vi "Main menu_4.vi"() -> ()   [LabVIEW 2021]
uses:
  <vilib>/event_ctls.llb/lveventtype.ctl
  <vilib>/Utility/file.llb/Write Delimited Spreadsheet (DBL).vi
panel:
  in  "Clear error":bool
  out "Error":bool
  out "Close":bool
  in  "?":T1(tab)
  in  "New_plot_window":bool
  in  "List of active windows":i32(listbox)
  in  "Close All plots":bool
  out "Trace_total samples":i32
  in  "CSV":bool
  in  "Start record":bool
  in  "Refresh \ntime (ms)":i32
  in  "Global Mode":enum32{"Item 0", "Item 1"}(radio)
  in  "Samples X Signal":u32
  in  "Trace names":string(combo)
  out "Signals":i32
  in  "CTRL enable":bool
  in  "Save CTRL parameters":bool
  out "Total\ncontrols":i32
  in  "# Control":string(combo)
  in  "CS enable":bool
  out "Current CS status":i32
  in  "CS_IF_Params":T2 {"CS_Duty" min=0 max=1}
  out "Connected":bool
  out "Saved":bool
  in  "Save conf":bool
  in  "Port":i32
  in  "hostname":string
  in  "timeout ms":i32
  in  "Send message":bool
  in  "Process":i32
  in  "msj":string
  out "error out":errorcluster
  # "ctrl_if:0\nctrl: 2\nset parm: 2"
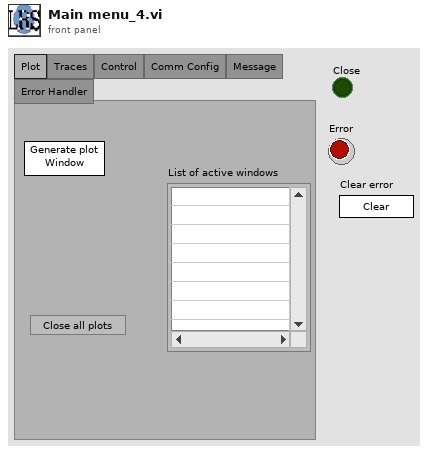
[diagram p1: front panel]
types:
  T1 = enum32{"Plot", "Traces", "Control", "Comm Config", "Message", "Error Handler"}
  T2 = cluster{"SET_PARAMETERS":i32, "CTLR":i32, "CS_Duty":sgl, "CTRL_IF_SET":i32}
  T3 = cluster{"Port":i32, "hostname":string, "status":bool, "timeout ms":i32, "TRACES_NAMES":string[], "Refresh time ms":i32, "Mode":enum32{"Item 0", "Item 1"}, "Start":bool, "DATA":sgl[][], "SIGNALS_NAMES":string[], "NB_SIGNALS":i32, "NB_TRACES":i32, "ID_TRACE":i32, "Mark":bool, "Counter":i32, "CTRLs_NAMES":string[], "NB_Ctrls":i32, "CS enable?":bool, "CS ID":i32}
  T4 = enum8{"Enabled", "Disabled", "Disabled and Grayed Out"}
  T5 = typedef "lveventtype.ctl" = enum32{"Null", "Timeout", "Annotation Menu Selection", "Annotation Menu Selection?", "App Instance Close", "App Instance Close?", "Autoscale Range Change", "Bookmark Info Change", "Cell Edit", "Cell Edit?", "Cursor Grab", "Cursor Grab?", "Cursor Menu Selection", "Cursor Menu Selection?", "Cursor Move", "Cursor Release", "Data Change", "Direction Change", "Display State Change", "Drag Ended", "Drag Enter", "Drag Leave", "Drag Over", "Drag Source Update", "Drag Starting", "Drag Starting?", "Drop", "Exec State Change", "Key Down", "Key Down?", "Key Repeat", "Key Repeat?", "Key Up", "Listbox Double Click", "Menu Activation?", "Menu Selection (App)", "Menu Selection? (App)", "Menu Selection (User)", "Mouse Down", "Mouse Down?", "Mouse Enter", "Mouse Leave", "Mouse Move", "Mouse Up", "Mouse Wheel", "NI Security User Change (App)", "Pane Size", "Panel Close", "Panel Close?", "Panel Resize", "Plot Attribute Change", "Scale Range Change", "Shortcut Menu Activation?", "Shortcut Menu Selection (App)", "Shortcut Menu Selection? (App)", "Shortcut Menu Selection (User)", "Tree Double Click", "Tree Drag", "Tree Drag?", "Tree Drop", "Tree Drop?", "Tree Item Close", "Tree Item Close?", "Tree Item Open", "Tree Item Open?", "User Event", "Value Change"}
  T6 = enum16{"open", "replace", "create", "open or create", "replace or create", "replace or create with confirmation"}
  T7 = enum32{"Invalid", "Standard", "Closed", "Hidden", "Minimized", "Maximized"}
  T8 = enum32{"invalid app kind", "Development System", "Run Time System", "Student Edition", "Embedded LabVIEW", "Evaluation", "Custom"}
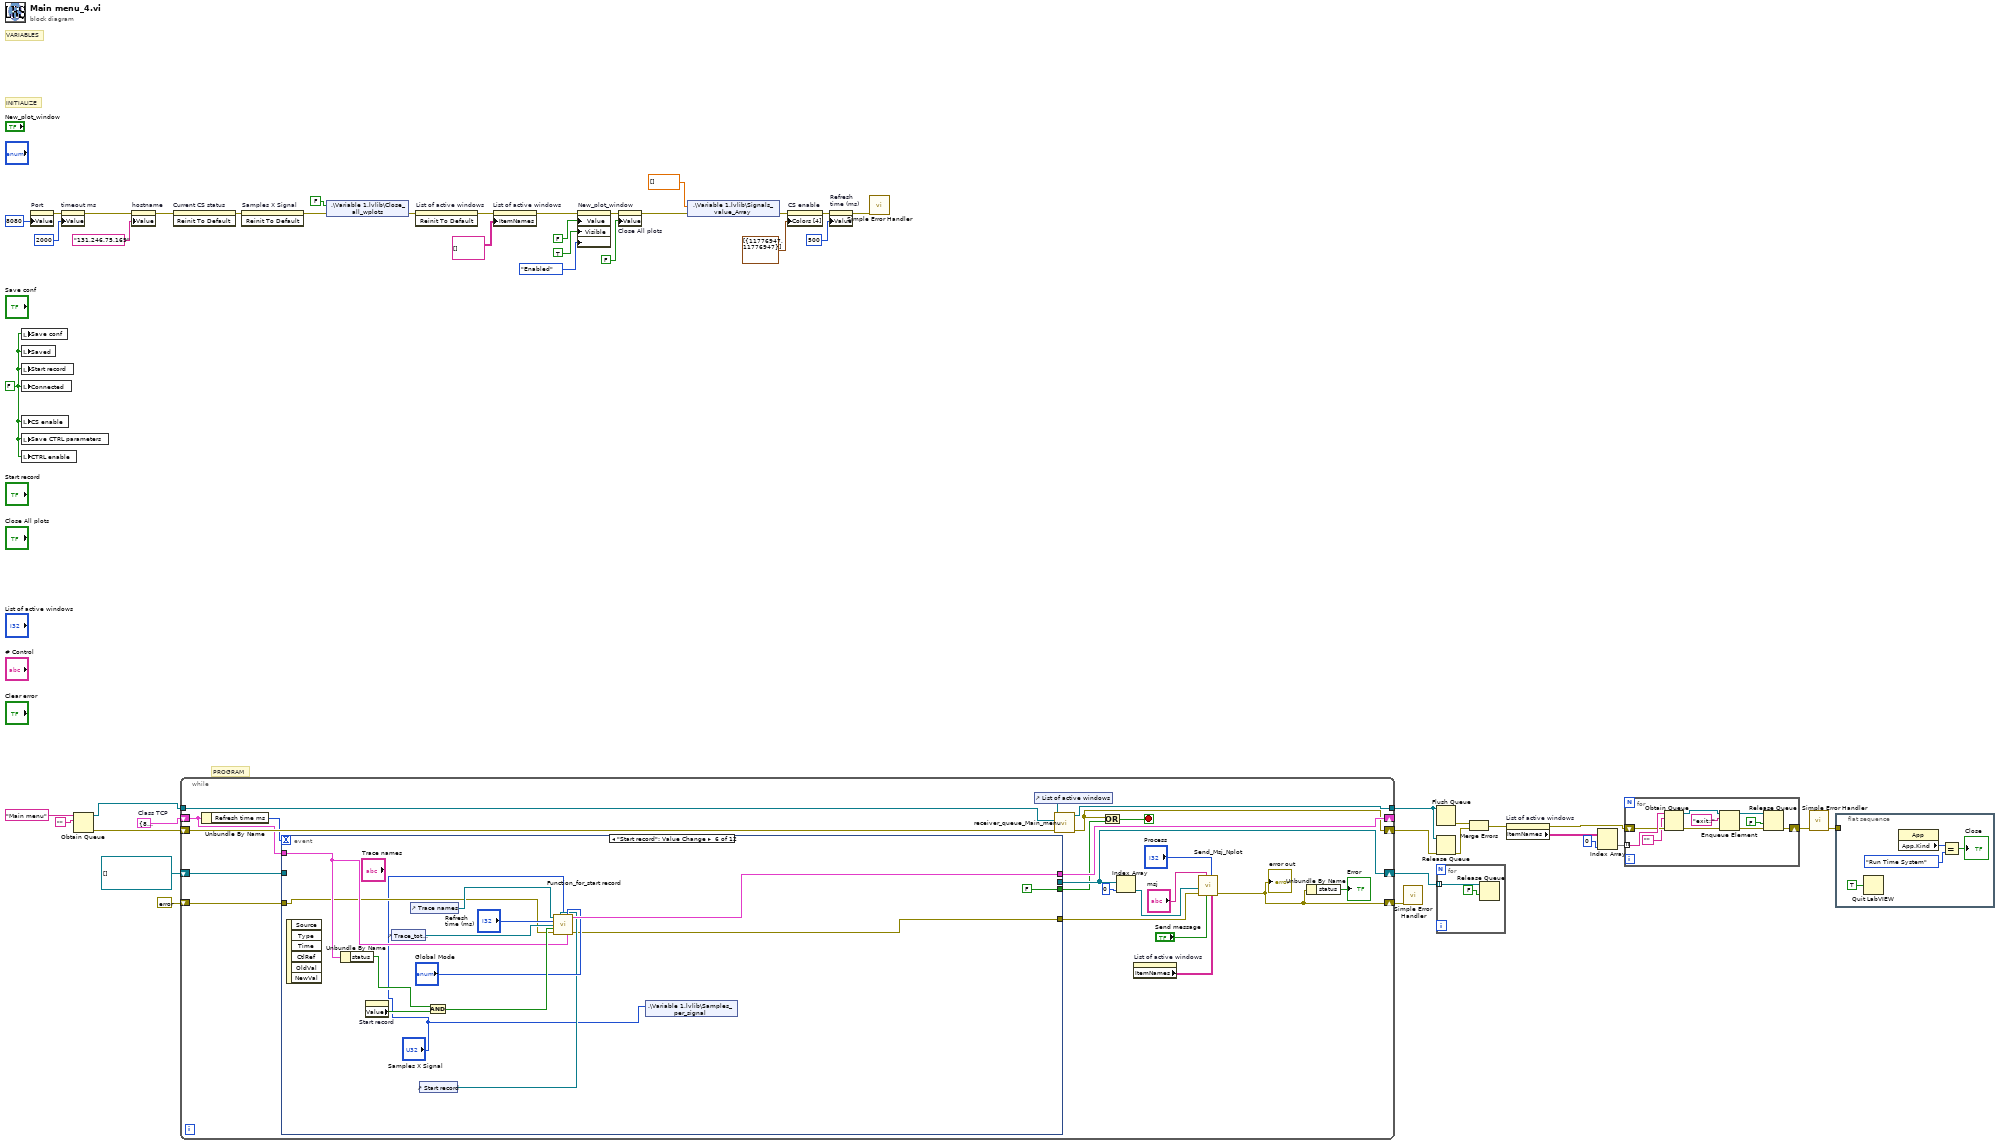
[diagram p0: block diagram]
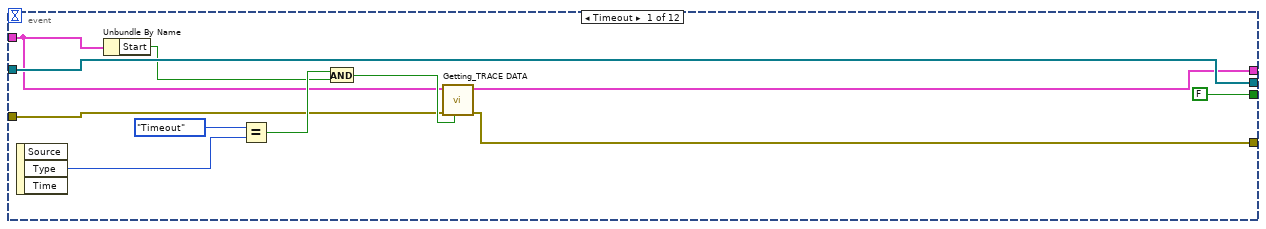
[diagram p2: hidden frame]
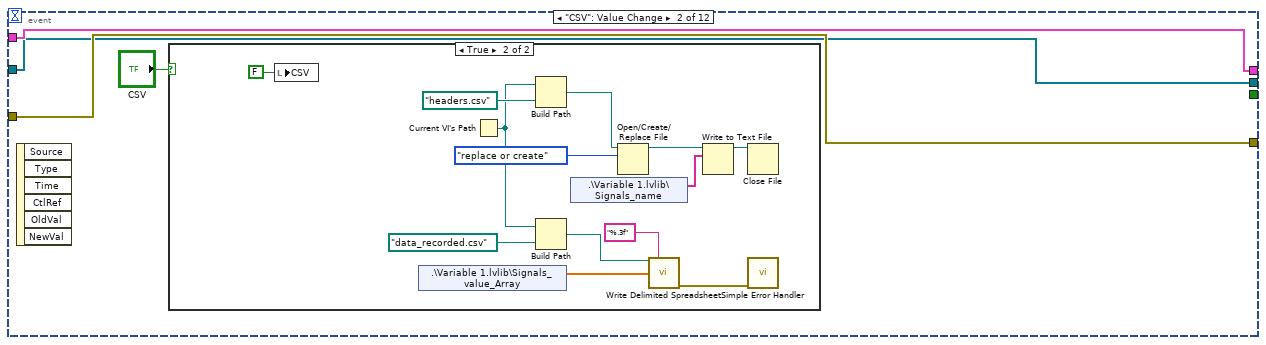
[diagram p3: hidden frame]
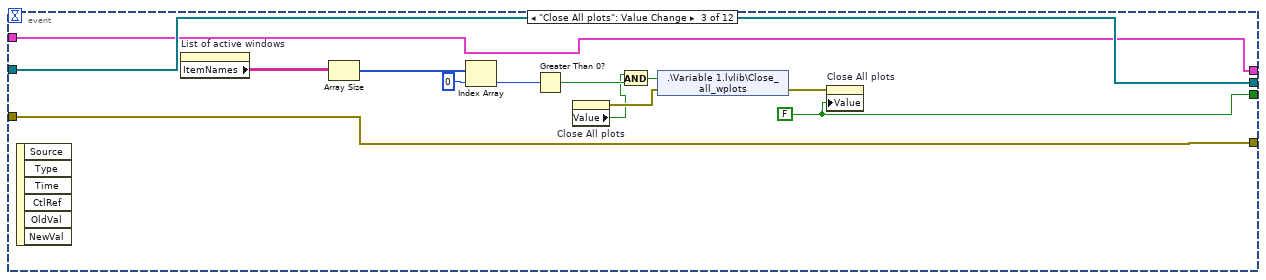
[diagram p5: hidden frame]
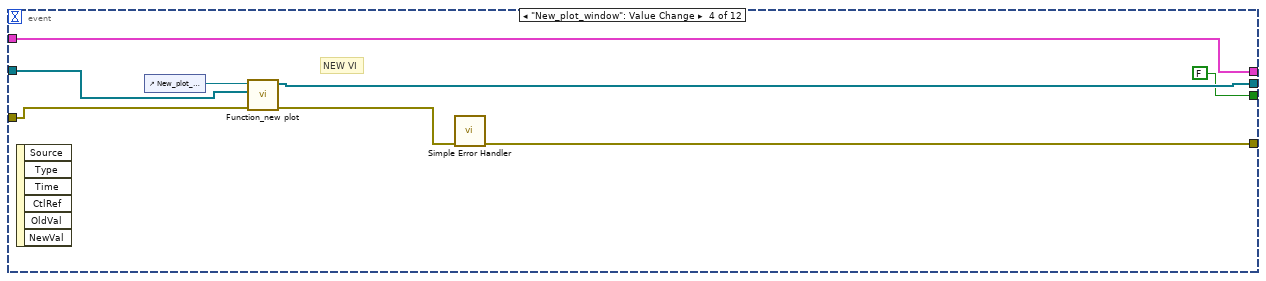
[diagram p6: hidden frame]
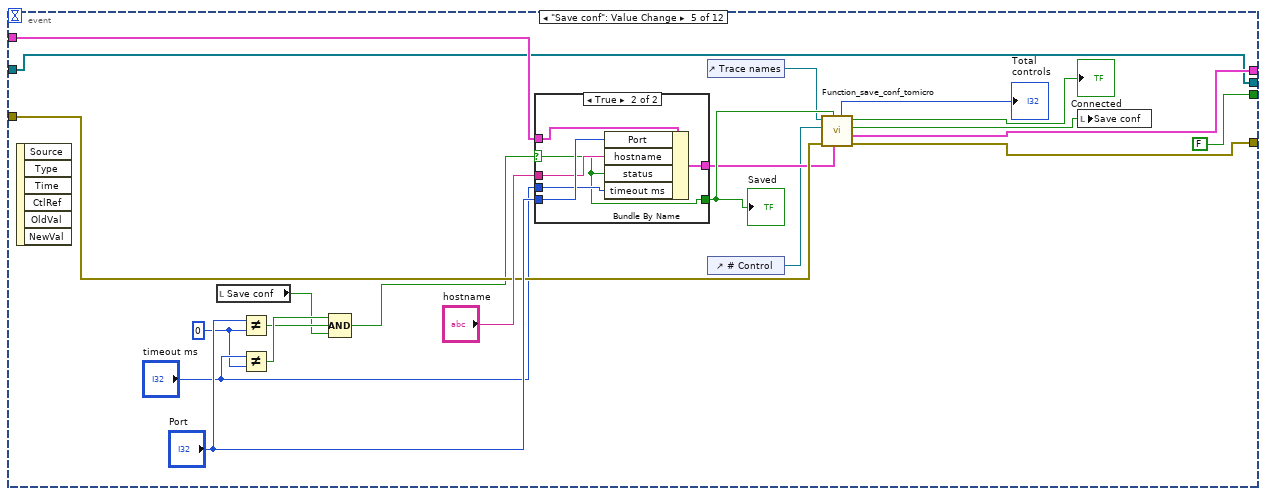
[diagram p7: hidden frame]
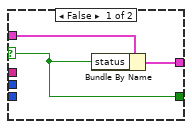
[diagram p8: hidden frame]
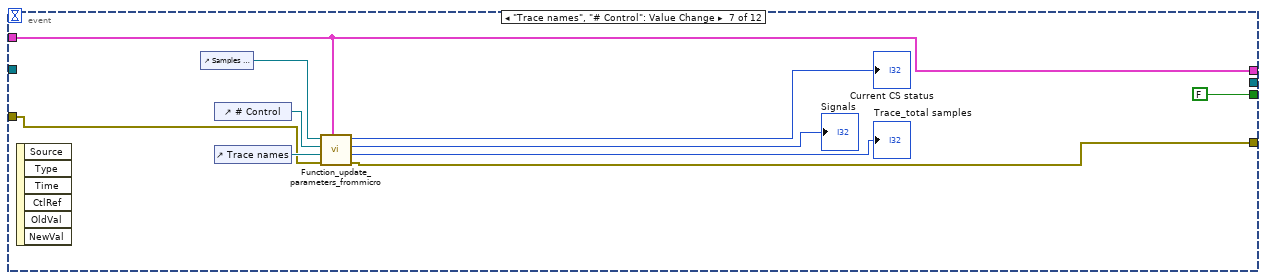
[diagram p9: hidden frame]
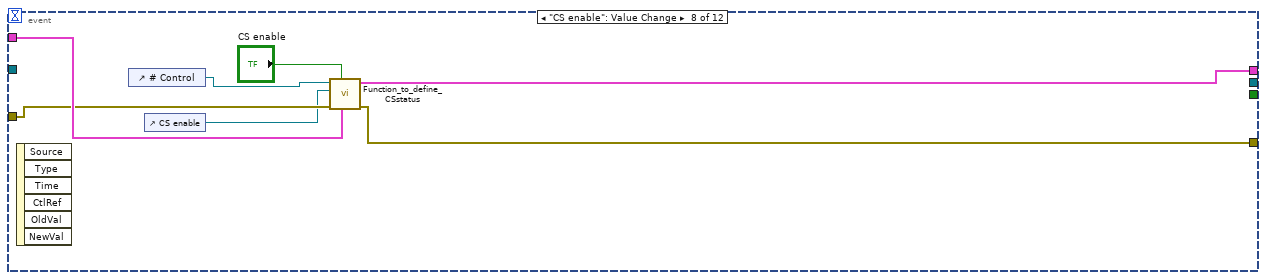
[diagram p10: hidden frame]
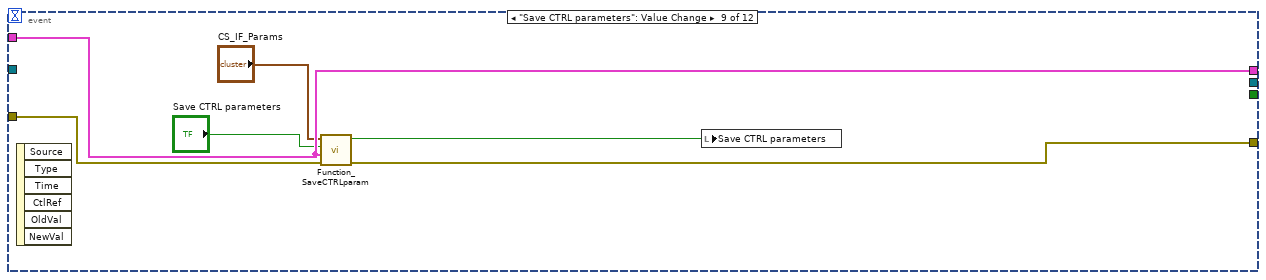
[diagram p11: hidden frame]
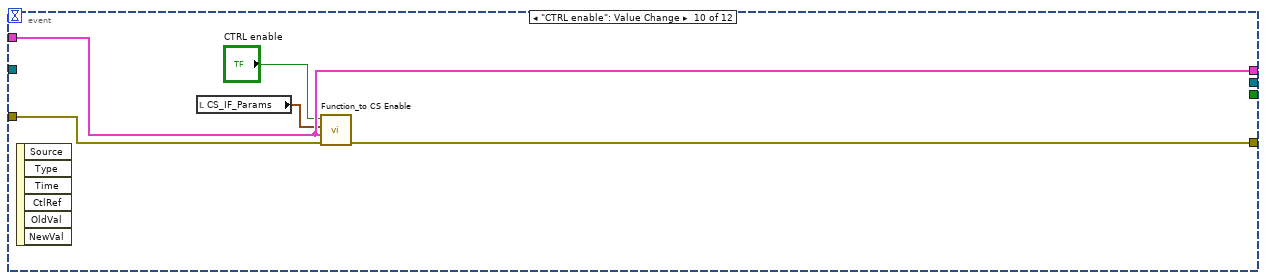
[diagram p12: hidden frame]
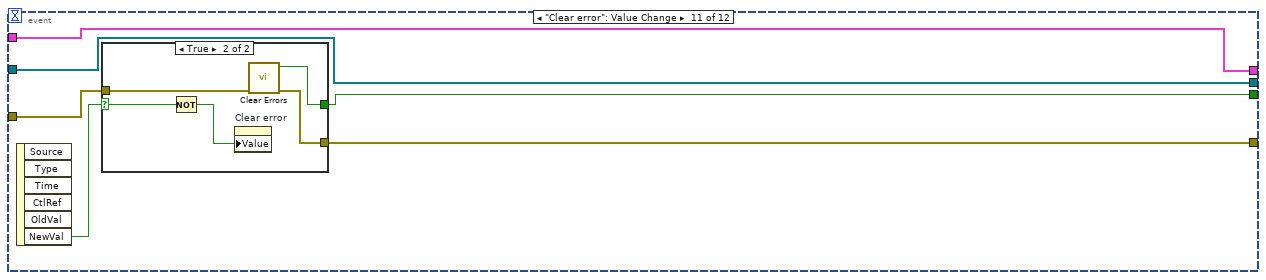
[diagram p13: hidden frame]
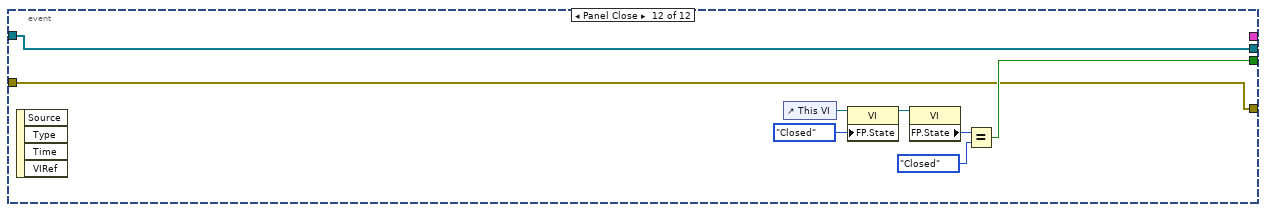
[diagram p15: hidden frame]
diagram:
  w26 = T3 {"Port"=8085, "hostname"="", "status"=FALSE, "timeout ms"=1000, "TRACES_NAMES"=[], "Refresh time ms"=500, "Mode"=enum."Item 0", "Start"=FALSE, "DATA"=[], "SIGNALS_NAMES"=[], "NB_SIGNALS"=0, "NB_TRACES"=0, "ID_TRACE"=0, "Mark"=FALSE, "Counter"=0, "CTRLs_NAMES"=[], "NB_Ctrls"=0, "CS enable?"=FALSE, "CS ID"=0}  # Class TCP
  w13 = FALSE ("Save conf")
  # "PROGRAM"
  # "INITIALIZE"
  # "VARIABLES"
  n1 = local write "Save conf"(w13) -> ()
  n2 = local write "Saved"(w13) -> ()
  n3 = local write "Start record"(w13) -> ()
  n4 = local write "Connected"(w13) -> ()
  n5 = local write "CS enable"(w13) -> ()
  n6 = local write "Save CTRL parameters"(w13) -> ()
  n7 = local write "CTRL enable"(w13) -> ()
  n8 = property on="Port" class="DigNum (strict)"("Value"=8080) -> (error out=w24:errorcluster)  [unwired: 2 in, 1 out]
  n9 = property on="timeout ms" class="DigNum (strict)"(error in=w24, "Value"=2000 ("timeout ms")) -> (error out=w20:errorcluster)  [unwired: 1 in, 1 out]
  n10 = Obtain Queue(name (unnamed)="Main menu", element data type="") -> (queue out=w39:refnum<queue>, error out=w37:errorcluster)  [unwired: 3 in, 1 out]
  n11 = property on="hostname" class="Str"(error in=w20, "Value"="131.246.75.169" ("hostname")) -> (error out=w7:errorcluster)  [unwired: 1 in, 1 out]
  n12 = invoke on="Current CS status" class="DigNum (strict)" method="Reinit To Default"(error in=w7) -> (error out=w18:errorcluster)  [unwired: 2 in, 2 out]
  n13 = while {
    shift-right: [w59] -> w43
    shift-left: refnum<queue>[] [] -> [w68]
    tunnel: w39 -> [w67]
    tunnel: [w66] -> w30
    shift-right: [w47] -> w38
    shift-left: w37 -> [w65]
    shift-right: [w64] -> _
    shift-left: w26 -> [w63]
    shift-right: [w52] -> w4
    shift-left: errorcluster {"status"=FALSE, "code"=0, "source"=""} ("error out") -> [w53]
    stop <- w48 stop-if-true
    n14 = Unbundle By Name(w63) -> ("Refresh time ms"=w57:i32)
    n15 = event shown="[5] \"Start record\": Value Change" {
      selector: _ -> [_ _ _ _ _ _ _ _ _ _ _ _]
      dyn-events: _ -> [_ _ _ _ _ _ _ _ _ _ _ _]
      timeout: w57 -> [_ _ _ _ _ _ _ _ _ _ _ _]
      tunnel: [FALSE ("f") _ w100 FALSE ("f") FALSE ("f") FALSE ("f") FALSE ("f") _ _ _ w192 w208] -> w49
      tunnel: [w79 w80 w109 w117 w118 _ _ _ _ _ w190 w207] -> w59
      tunnel: w68 -> [w79 w80 w109 w116 w118 _ _ _ _ _ w190 w207]
      tunnel: [w72 w82 w104 w114 w131 w158 w170 w178 w183 w188 w191 _] -> w64
      tunnel: w63 -> [w73 w82 w104 w114 w138 w159 w170 w177 w183 w188 w191 _]
      tunnel: w53 -> [w70 w81 w103 w112 w134 w150 w163 w174 w184 w189 w194 w206]
      tunnel: [w69 w81 w103 w110 w119 w149 w162 w172 w179 w185 w193 w206] -> w50
      event Timeout {
        n16 = event-data() -> ("Type"=w77:T5)  [unwired: 1 in, 2 out]
        n17 = Unbundle By Name(w73) -> ("Start"=w75:bool)
        n18 = Equal?(x=lveventtype."Timeout" ("Type"), y=w77) -> (x = y?=w76:bool)
        n19 = And(x=w76, y=w75) -> (x .and. y?=w74:bool)
        n20 = call "Getting_TRACE DATA.vi"("Start+timeout?"=w74, "error in (no error)"=w70, "Class TCP in"=w73) -> ("error out"=w69:errorcluster, "Class TCP out"=w72:T3)  [unwired: 7 in]
      }
      event "CSV": Value Change {
        n21 = event-data() -> ()  [unwired: 1 in, 6 out]
        n22 = case shown="True" "CSV" {
          frame False {
          }
          frame True {
            n23 = local write "CSV"(FALSE ("CSV")) -> ()
            n24 = shared-variable ".\\Variable 1.lvlib\\Signals_value_Array"() -> (w93:dbl[])  [unwired: 1 in, 1 out]
            n25 = Current VI's Path() -> (path=w84:path)
            n26 = Build Path(base path=w84, name or relative path=path "headers.csv") -> (appended path=w90:path)
            n27 = Build Path(base path=w84, name or relative path=path "data_recorded.csv") -> (appended path=w92:path)
            n28 = shared-variable ".\\Variable 1.lvlib\\Signals_name"() -> (w87:string[])  [unwired: 1 in, 1 out]
            n29 = Open/Create/Replace File(file path (use dialog)=w90, operation (0:open)=T6."replace or create") -> (refnum out=w88:refnum<file>)  [unwired: 4 in, 2 out]
            n30 = call-poly <vilib>:"Write Delimited Spreadsheet.vi"("file path (dialog if empty)"=w92, "format (%.3f)"="%.3f", "1D data"=w93) -> ("error out"=w94:errorcluster)  [unwired: 11 in, 1 out]
            n31 = Write to Text File(file (use dialog)=w88, text=w87) -> (refnum out=w86:refnum<file>)  [unwired: 2 in, 2 out]
            n32 = Close File(refnum=w86) -> ()  [unwired: 1 in, 2 out]
            n33 = call <vilib>:"Simple Error Handler.vi"("error in (no error)"=w94) -> ()  [unwired: 4 in, 5 out]
          }
        }
      }
      event "Close All plots": Value Change {
        w100 = FALSE ("f")
        n34 = event-data() -> ()  [unwired: 1 in, 6 out]
        n35 = property on="List of active windows" class="MCListbox (strict)"() -> ("ItemNames"=w105:string[][])  [unwired: 2 in, 2 out]
        n36 = Array Size(array=w105) -> (size(s)=w108:i32[])
        n37 = Index Array(array=w108, index=0) -> (element=w106:i32)
        n38 = Greater Than 0?(x=w106) -> (x > 0?=w99:bool)
        n39 = property on="Close All plots" class="Bool (strict)"() -> (error out=w98:errorcluster, "Value"=w97:bool)  [unwired: 2 in, 1 out]
        n40 = And(x=w97, y=w99) -> (x .and. y?=w102:bool)
        n41 = shared-variable ".\\Variable 1.lvlib\\Close_all_wplots"(w102, error in=w98) -> (error out=w101:errorcluster)
        n42 = property on="Close All plots" class="Bool (strict)"(error in=w101, "Value"=w100) -> ()  [unwired: 1 in, 2 out]
      }
      event "New_plot_window": Value Change {
        # "NEW VI"
        n43 = event-data() -> ()  [unwired: 1 in, 6 out]
        n44 = control-ref of="New_plot_window"() -> (w113:refnum<vi>)
        n45 = call "Function_new plot.vi"("error in (no error)"=w112, "Array in"=w116, "Boolean in"=w113) -> ("error out"=w111:errorcluster, "Array out"=w117:refnum<queue>[])  [unwired: 7 in]
        n46 = call <vilib>:"Simple Error Handler.vi"("error in (no error)"=w111) -> ("error out"=w110:errorcluster)  [unwired: 4 in, 4 out]
      }
      event "Save conf": Value Change {
        w120 = 0 ("y")
        n47 = event-data() -> ()  [unwired: 1 in, 6 out]
        n48 = local read "Save conf"() -> (w122:bool)
        n49 = Not Equal?(x="Port", y=w120) -> (x != y?=w123:bool)
        n50 = Not Equal?(x="timeout ms", y=w120) -> (x != y?=w124:bool)
        n51 = Compound Arithmetic op=AND(w124, w123, w122) -> (w121:bool)
        n52 = case shown="True" w121 {
          selector: w121 -> [w139 w142]
          tunnel: [w139 w142] -> w135
          tunnel: "Port" -> [_ w146]
          tunnel: "hostname" -> [_ w145]
          tunnel: [w141 w144] -> w132
          tunnel: w138 -> [w140 w147]
          tunnel: "timeout ms" -> [_ w143]
          frame False {
            n53 = Bundle By Name(cluster=w140, "status"=w139) -> (w141:T3)
          }
          frame True {
            n54 = Bundle By Name(cluster=w147, "Port"=w146, "hostname"=w145, "status"=w142, "timeout ms"=w143) -> (w144:T3)
          }
        }
        "Saved" <- w135
        n55 = control-ref of="Trace names"() -> (w126:refnum<vi>)
        n56 = control-ref of="# Control"() -> (w125:refnum<vi>)
        n57 = call "Function_save_conf_tomicro.vi"("Class TCP in"=w132, "Saved configuration?"=w135, "error in (no error)"=w134, "CmbBox Refnum in"=w125, "ComboBox in"=w126) -> ("error out"=w119:errorcluster, "Class TCP out"=w131:T3, "Save conf?"=w133:bool, "Connected?"=→"Connected":bool, "NB_CSs"=→"Total\ncontrols":i32)  [unwired: 2 in]
        n58 = local write "Save conf"(w133) -> ()
      }
      event "Start record": Value Change {
        n59 = event-data() -> ()  [unwired: 1 in, 6 out]
        n60 = Unbundle By Name(w159) -> ("status"=w161:bool)
        n61 = property on="Start record" class="Bool (strict)"() -> ("Value"=w156:bool)  [unwired: 2 in, 2 out]
        n62 = control-ref of="Trace_total samples"() -> (w151:refnum<vi>)
        n63 = control-ref of="Trace names"() -> (w153:refnum<vi>)
        n64 = control-ref of="Start record"() -> (w152:refnum<vi>)
        n65 = And(x=w161, y=w156) -> (x .and. y?=w160:bool)
        n66 = call "Function_for_start record.vi"("Trace names"=w153, "Start record?"=w152, "Samples X Signal"="Samples X Signal", "Global Mode"="Global Mode", "Refresh \ntime (ms)"="Refresh \ntime (ms)", "total samples?"=w151, "status+start record"=w160, "error in (no error)"=w150, "Class TCP in"=w159) -> ("Class TCP out"=w158:T3, "error out"=w149:errorcluster)  [unwired: 5 in]
        n67 = shared-variable ".\\Variable 1.lvlib\\Samples_per_signal"("Samples X Signal") -> ()  [unwired: 1 in, 1 out]
      }
      event "Trace names", "# Control": Value Change {
        n68 = event-data() -> ()  [unwired: 1 in, 6 out]
        n69 = control-ref of="Samples X Signal"() -> (w166:refnum<vi>)
        n70 = control-ref of="# Control"() -> (w165:refnum<vi>)
        n71 = control-ref of="Trace names"() -> (w164:refnum<vi>)
        n72 = call "Function_update_parameters_frommicro.vi"("Class TCP"=w170, "error in (no error)"=w163, "Trace names"=w164, "# Control"=w165, "SamplesXSignal?"=w166) -> ("error out"=w162:errorcluster, "TRACE_SIZE"=→"Trace_total samples":i32, "NB_TRACED_SIGNALS"=→"Signals":i32, "CS STATUS"=→"Current CS status":i32)  [unwired: 3 in]
      }
      event "CS enable": Value Change {
        n73 = event-data() -> ()  [unwired: 1 in, 6 out]
        n74 = control-ref of="# Control"() -> (w175:refnum<vi>)
        n75 = control-ref of="CS enable"() -> (w173:refnum<vi>)
        n76 = call "Function_to_define_CSstatus.vi"("Class TCP in"=w177, 7:"CS enable"="CS enable", "error in (no error)"=w174, 10:"CS enable"=w173, "# Control?"=w175) -> ("error out"=w172:errorcluster, "Class TCP out"=w178:T3)  [unwired: 5 in]
      }
      event "Save CTRL parameters": Value Change {
        n77 = event-data() -> ()  [unwired: 1 in, 6 out]
        n78 = call "Function_SaveCTRLparam.vi"("error in (no error)"=w184, "Class TCP"=w183, "Save CTRL params"="Save CTRL parameters", "CS_IF_Params"="CS_IF_Params") -> ("error out"=w179:errorcluster, "Saved CTRL params ?"=w180:bool)  [unwired: 6 in]
        n79 = local write "Save CTRL parameters"(w180) -> ()
      }
      event "CTRL enable": Value Change {
        n80 = event-data() -> ()  [unwired: 1 in, 6 out]
        n81 = local read "CS_IF_Params"() -> (w186:T2)
        n82 = call "Function_to CS Enable.vi"("error in (no error)"=w189, "Class TCP"=w188, "CS_IF_Params"=w186, "CTRL enable"="CTRL enable") -> ("error out"=w185:errorcluster)  [unwired: 7 in]
      }
      event "Clear error": Value Change {
        n83 = event-data() -> ("NewVal"=w195:bool)  [unwired: 1 in, 5 out]
        n84 = case shown="True" w195 {
          selector: w195 -> [w196 w200]
          tunnel: w194 -> [w197 w202]
          tunnel: [w197 w201] -> w193
          tunnel: [w196 w198] -> w192
          frame False {
          }
          frame True {
            n85 = Not(x=w200) -> (.not. x?=w199:bool)
            n86 = property on="Clear error" class="Bool (strict)"("Value"=w199) -> ()  [unwired: 2 in, 2 out]
            n87 = call <vilib>:"Clear Errors.vi"("error in (no error)"=w202) -> ("error out"=w201:errorcluster, "specific error cleared?"=w198:bool)  [unwired: 5 in]
          }
        }
      }
      event Panel Close {
        n88 = event-data() -> ()  [unwired: 1 in, 4 out]
        n89 = control-ref of="This VI"() -> (w205:refnum<vi>)
        n90 = property class="VI"(reference=w205, "FP.State"=T7."Closed" ("Front Panel Window:State")) -> (reference out=w204:refnum<vi>)  [unwired: 1 in, 1 out]
        n91 = property class="VI"(reference=w204) -> ("FP.State"=w210:T7)  [unwired: 1 in, 2 out]
        n92 = Equal?(x=w210, y=T7."Closed") -> (x = y?=w208:bool)
      }
    }
    n93 = control-ref of="List of active windows"() -> (w56:refnum<vi>)
    n94 = call "receiver_queue_Main_menu.vi"("error in (no error)"=w65, "queue in"=w67, "MulticolumnListbox in"=w56) -> ("error out"=w47:errorcluster, "Queue out"=w66:refnum<queue>)  [unwired: 7 in]
    n95 = Or(x=w47, y=w49) -> (x .or. y?=w48:bool)
    n96 = Index Array(array=w59, index=0) -> (element=w58:refnum<queue>)
    n97 = property on="List of active windows" class="MCListbox (strict)"() -> ("ItemNames"=w61:string[][])  [unwired: 2 in, 2 out]
    n98 = call "Send_Msj_Nplot.vi"("ItemNames"=w61, "Process in"="Process", "Send message"="Send message", "msj"="msj", "error in (no error)"=w50, "queue in"=w58) -> ("error out"=w52:errorcluster)  [unwired: 5 in]
    "error out" <- w52
    n99 = Unbundle By Name(w52) -> ("status"=→"Error":bool)
  }
  n100 = invoke on="Samples X Signal" class="DigNum (strict)" method="Reinit To Default"(error in=w18) -> (error out=w17:errorcluster)  [unwired: 2 in, 2 out]
  n101 = shared-variable ".\\Variable 1.lvlib\\Close_all_wplots"(FALSE ("Close_all_wplots"), error in=w17) -> (error out=w23:errorcluster)
  n102 = invoke on="List of active windows" class="MCListbox (strict)" method="Reinit To Default"(error in=w23) -> (error out=w28:errorcluster)  [unwired: 2 in, 2 out]
  n103 = property on="List of active windows" class="MCListbox (strict)"(error in=w28, "ItemNames"=string[][] [] ("Item Names")) -> (error out=w16:errorcluster)  [unwired: 1 in, 1 out]
  n104 = property on="New_plot_window" class="Bool (strict)"(error in=w16, "Value"=FALSE ("New plot"), "Visible"=TRUE, "DisabledEnum"=T4."Enabled" ("Disabled")) -> (error out=w15:errorcluster)  [unwired: 1 in, 1 out]
  n105 = property on="Close All plots" class="Bool (strict)"(error in=w15, "Value"=FALSE ("Cancel Button")) -> (error out=w6:errorcluster)  [unwired: 1 in, 1 out]
  n106 = shared-variable ".\\Variable 1.lvlib\\Signals_value_Array"(dbl[] [] ("Signals_value_Array"), error in=w6) -> (error out=w12:errorcluster)
  n107 = property on="CS enable" class="Bool (strict)"(error in=w12, "Colors [4]"=cluster{u32, u32}[] [{11776947, 11776947}]) -> (error out=w10:errorcluster)  [unwired: 1 in, 1 out]
  n108 = property on="Refresh \ntime (ms)" class="DigNum (strict)"(error in=w10, "Value"=500 ("Refresh \ntime (ms)")) -> (error out=w9:errorcluster)  [unwired: 1 in, 1 out]
  n109 = call <vilib>:"Simple Error Handler.vi"("error in (no error)"=w9) -> ()  [unwired: 4 in, 5 out]
  n110 = call <vilib>:"Simple Error Handler.vi"("error in (no error)"=w4) -> ()  [unwired: 4 in, 5 out]
  n111 = Flush Queue(queue=w30) -> (error out=w3:errorcluster)  [unwired: 1 in, 2 out]
  n112 = Release Queue(queue=w30, error in (no error)=w38) -> (error out=w2:errorcluster)  [unwired: 1 in, 2 out]
  n113 = for {
    tunnel: w43 -> [w212] mode=indexing
    n114 = Release Queue(queue=w212, force destroy? (F)=FALSE) -> ()  [unwired: 1 in, 3 out]
  }
  n115 = Merge Errors(w3, w2) -> (w1:errorcluster)
  n116 = property on="List of active windows" class="MCListbox (strict)"(error in=w1) -> (error out=w33:errorcluster, "ItemNames"=w36:string[][])  [unwired: 1 in, 1 out]
  n117 = Index Array(array=w36, index (col)=0 ("disabled index (col)")) -> (element=w34:string[])  [unwired: 1 in]
  n118 = for {
    tunnel: w34 -> [w222] mode=indexing
    shift-right: [w219] -> w32
    shift-left: w33 -> [w221]
    n119 = Obtain Queue(name (unnamed)=w222, element data type="", error in (no error)=w221) -> (queue out=w214:refnum<queue>, error out=w216:errorcluster)  [unwired: 2 in, 1 out]
    n120 = Enqueue Element(queue=w214, element="exit::", error in (no error)=w216) -> (queue out=w213:refnum<queue>, error out=w215:errorcluster)  [unwired: 1 in, 1 out]
    n121 = Release Queue(queue=w213, force destroy? (F)=FALSE, error in (no error)=w215) -> (error out=w219:errorcluster)  [unwired: 2 out]
  }
  n122 = call <vilib>:"Simple Error Handler.vi"("error in (no error)"=w32) -> ("error out"=w31:errorcluster)  [unwired: 4 in, 4 out]
  n123 = flat-sequence {
    tunnel: w31 -> [_]
    frame #0 {
      n124 = Quit LabVIEW(quit? (T)=TRUE) -> ()
      n125 = property class="App"() -> ("App.Kind"=w226:T8)  [unwired: 2 in, 2 out]
      n126 = Equal?(x=w226, y=T8."Run Time System" ("Application:Kind")) -> (x = y?=→"Close":bool)
    }
  }
